vi "Set_WCM_limits.vi"(8 "error in (no error)":errorcluster, 11 "Control-Client in":refnum<class "Control-Client.lvclass">) -> (0 "error out":errorcluster, 3 "Control-Client out":refnum<class "Control-Client.lvclass">)   [LabVIEW 2019, in "Control-Client.lvclass"]
uses:
  Control-Client.lvclass
  Control-Client.lvclass/Control-Client.ctl
  Experiments/Experiment.lvclass
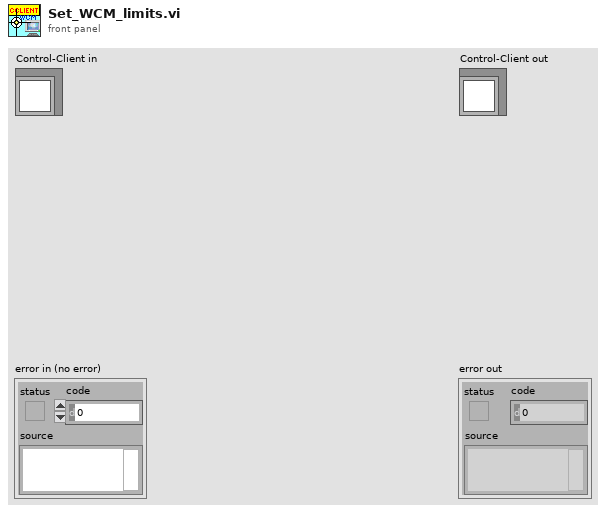
[diagram p1: front panel]
types:
  T1 = cluster{"WCM_min":dbl, "WCM_max":dbl, "WCM_value":dbl}
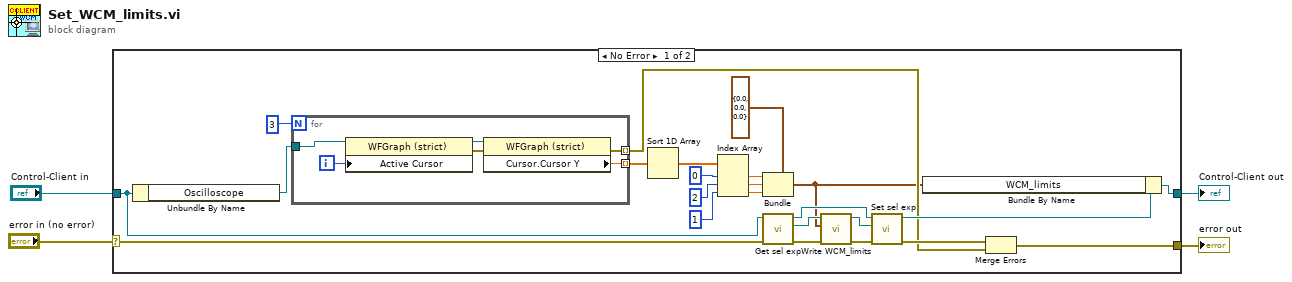
[diagram p0: block diagram]
diagram:
  n1 = case shown="No Error" "error in (no error)" {
    selector: "error in (no error)" -> [w27 w36]
    tunnel: [w22 w36] -> w3
    tunnel: [w19 w35] -> w1
    tunnel: "Control-Client in" -> [w28 w35]
    frame No Error {
      n2 = Unbundle By Name(w28) -> ("Oscilloscope"=w17:refnum<vi>)
      n3 = for {
        N: 3 -> [_]
        tunnel: [w31] -> w15 mode=indexing
        tunnel: w17 -> [w30]
        tunnel: [w29] -> w6 mode=indexing
        i -> [w32]
        n4 = property class="WFGraph (strict)"(reference=w30, "Active Cursor"=w32) -> (reference out=w34:refnum<vi>, error out=w33:errorcluster)  [unwired: 1 in]
        n5 = property class="WFGraph (strict)"(reference=w34, error in=w33) -> (error out=w29:errorcluster, "Cursor.Cursor Y"=w31:dbl)  [unwired: 1 out]
      }
      n6 = Sort 1D Array(array=w15) -> (sorted array=w14:dbl[])
      n7 = Index Array(array=w14, index #1=0 ("index"), index #2=2 ("index"), index #3=1 ("index")) -> (element #1=w10:dbl, element #2=w9:dbl, element #3=w8:dbl)
      n8 = Bundle(cluster=T1 {"WCM_min"=0.0, "WCM_max"=0.0, "WCM_value"=0.0} ("WCM_limits"), "WCM_min"=w10, "WCM_max"=w9, "WCM_value"=w8) -> (w5:T1)
      n9 = call "Get sel exp.vi"("error in (no error)"=w27, "Control-Client in"=w28) -> ("error out"=w26:errorcluster, "Sel experiment"=w23:refnum<class "Experiment.lvclass">, "Control-Client out"=w21:refnum<class "Control-Client.lvclass">)  [unwired: 7 in]
      n10 = call-dynamic "Write WCM_limits.vi"("error in (no error)"=w26, "WCM_limits"=w5, "Experiment in"=w23) -> ("error out"=w25:errorcluster, "Experiment out"=w24:refnum<class "Experiment.lvclass">)  [unwired: 7 in]
      n11 = call "Set sel exp.vi"("error in (no error)"=w25, "Experiment"=w24, "Control-Client in"=w21) -> ("error out"=w7:errorcluster, "Control-Client out"=w20:refnum<class "Control-Client.lvclass">)  [unwired: 7 in]
      n12 = Bundle By Name(cluster=w20, "WCM_limits"=w5) -> (w19:refnum<class "Control-Client.lvclass">)
      n13 = Merge Errors(w7, w6) -> (w22:errorcluster)
    }
    frame Error {
    }
  }
  "error out" <- w3
  "Control-Client out" <- w1
